vi "Waiting for All Active ActorRef.vi"(8 "Error In":errorcluster, 11 "Core In":refnum<class "Core.lvclass">) -> (0 "Error Out":errorcluster, 2 "Timeout":bool, 3 "Core Out":refnum<class "Core.lvclass">)   [LabVIEW 2019, in "Core.lvlib" / "Core.lvclass"]
uses:
  Core.lvclass
  C:/Projekty/_Wewnetrzne/PC_ActorFramework/07_Program/LABVIEW/02_Source/Modules/ModuleAbstract/ModuleAbstract.lvclass
  ModuleAbstract/ModuleAbstract.lvclass/ModuleAbstract.ctl
  Core.lvclass/Core.ctl
  Containers/ActorRefContainer/ActorRefContainer.lvclass
  ModuleAbstract/ModuleAbstract.lvclass
  C:/Program Files (x86)/National Instruments/LabVIEW 2019/vi.lib/ActorFramework/Actor/Actor.lvclass
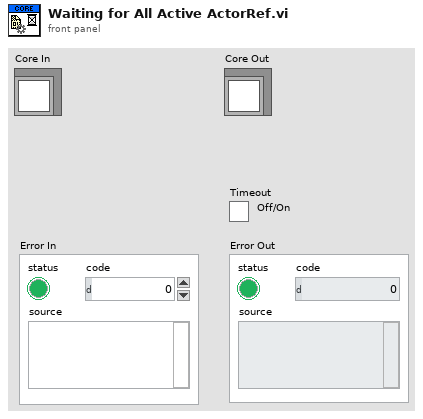
[diagram p1: front panel]
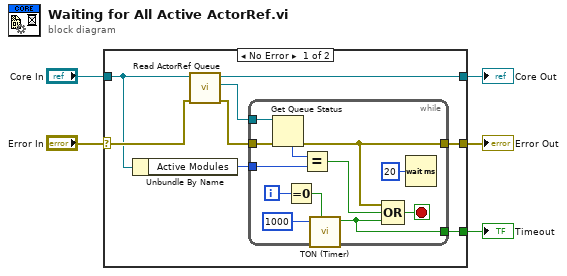
[diagram p0: block diagram]
diagram:
  n1 = case shown="No Error" "Error In" {
    selector: "Error In" -> [w9 w27]
    tunnel: [w13 _] -> w5
    tunnel: [w12 w27] -> w4
    tunnel: "Core In" -> [w7 w26]
    tunnel: [w11 w26] -> w1
    frame No Error {
      n2 = Unbundle By Name(w7) -> ("Active Modules"=w6:i32)
      n3 = call "Read ActorRef Queue.vi"("error in (no error)"=w9, "ModuleAbstract in"=w7) -> ("error out"=w8:errorcluster, "ActorRef Queue"=w10:refnum<queue>, "ModuleAbstract out"=w11:refnum<class "Core.lvclass">)  [unwired: 7 in]
      n4 = while {
        tunnel: w10 -> [w25]
        tunnel: w8 -> [w24]
        tunnel: w6 -> [w14]
        tunnel: [w16] -> w13
        tunnel: [w15] -> w12
        i -> [w20]
        stop <- w17 stop-if-true
        n5 = Get Queue Status(queue=w25, error in (no error)=w24) -> (error out=w15:errorcluster, # elements in queue=w23:i32)  [unwired: 1 in, 6 out]
        n6 = Equal To 0?(x=w20) -> (x = 0?=w19:bool)
        n7 = Equal?(x=w23, y=w14) -> (x = y?=w18:bool)
        n8 = call "TON (Timer).vi"("Reset"=w19, "Set Time"=u32 1000) -> ("Timeout"=w16:bool)  [unwired: 7 in, 2 out]
        n9 = Compound Arithmetic op=OR(w15, w18, w16) -> (w17:bool)
        n10 = Wait (ms)(milliseconds to wait=u32 20) -> ()  [unwired: 1 out]
      }
    }
    frame Error {
    }
  }
  "Timeout" <- w5
  "Error Out" <- w4
  "Core Out" <- w1
